vi "JKISM++ List Modules.vi"(8 "Error in":errorcluster caption="Error in (no error)") -> (0 "Error out":errorcluster, 3 "Name":string[](array[string]))   [LabVIEW 2014, in "JKI-State-Machine-Plus.lvlib"]
uses:
  JKI-State-Machine-Plus.lvlib
  _Support/_JKISMQFGVOPER.ctl
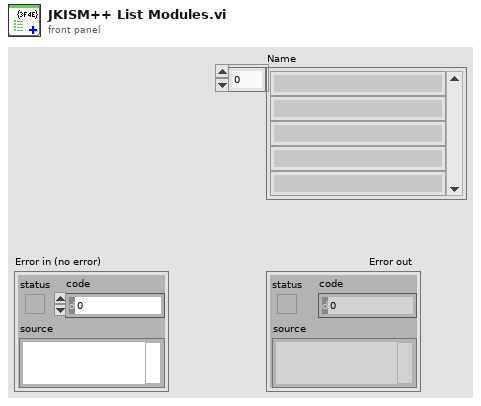
[diagram p1: front panel]
types:
  T1 = typedef "JKI-State-Machine-Plus.lvlib/_JKISMQFGVOPER.ctl" = enum16{"Get By Name", "List", "Check If Name Exists", "Release"}
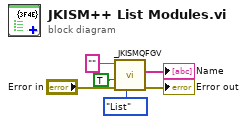
[diagram p0: block diagram]
diagram:
  n1 = call "_JKISMQFGV.vi"(6:_JKISMQFGVOPER."List", "Error in"="Error in", "create if not found? (T)"=TRUE, "Name(\"\" to use uuid) in"="" ("Name(\"\" to use uuid) in")) -> ("Error out"=→"Error out":errorcluster, "Name"=→"Name":string[])  [unwired: 4 in, 2 out]
